vi "绝对时间图表.vi"() -> ()   [LabVIEW 2012]
panel:
  in  "stop":bool
  in  "每秒采样数":dbl=15.0
  out "随机数波形图表":dbl(graph)=-0.7727644875559871
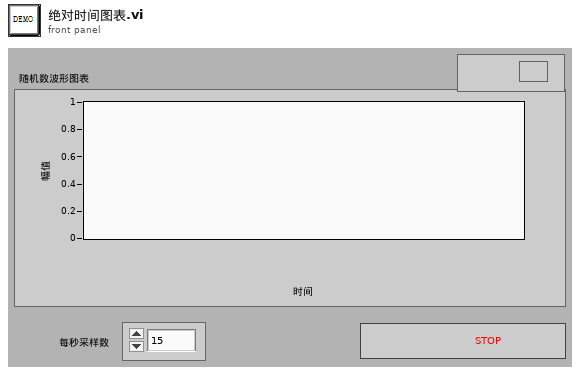
[diagram p1: front panel]
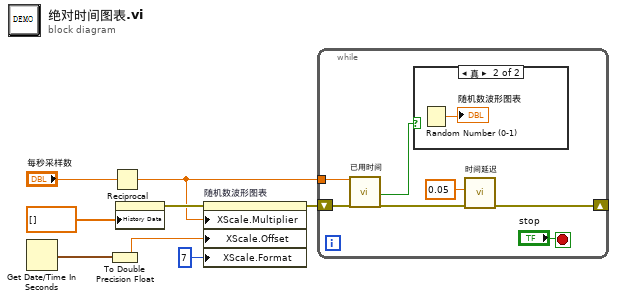
[diagram p0: block diagram]
diagram:
  n1 = Get Date/Time In Seconds() -> (seconds since 1Jan1904=w7:timestamp)
  n2 = To Double Precision Float(number=w7) -> (double precision float=w8:dbl)
  n3 = Reciprocal(x="每秒采样数") -> (1/x=w1:dbl)
  n4 = property on="随机数波形图表" class="WFChart (严格)"("History Data"=dbl[] []) -> (error out=w3:errorcluster)  [unwired: 2 in, 1 out]
  n5 = property on="随机数波形图表" class="WFChart (严格)"(error in=w3, "XScale.Multiplier"=w1, "XScale.Offset"=w8, "XScale.Format"=u8 7 ("X Scale.Display Format:Format")) -> (error out=w5:errorcluster)  [unwired: 1 in, 1 out]
  n6 = while {
    tunnel: w1 -> [w14]
    shift-right: [w10] -> _
    shift-left: w5 -> [w12]
    stop <- "stop" stop-if-true
    n7 = call "已用时间"("Time Target (s)"=w14, "error in (no error)"=w12) -> ("Time has Elapsed"=w13:bool, "error out"=w11:errorcluster)  [unwired: 10 in, 6 out]
    n8 = case shown="真" w13 {
      frame False {
      }
      frame True {
        n9 = Random Number (0-1)() -> (number: 0 to 1=→"随机数波形图表":dbl)
      }
    }
    n10 = call "时间延迟"("error in (no error)"=w11, "Delay Time (s)"=0.05) -> ("error out"=w10:errorcluster)  [unwired: 9 in]
  }
